vi "Eurotherm set.vi"(8 "error in":errorcluster, 10 "SP&CRC":u8[](array[numeric])=[65, 32, 0, 0, 133, 120], 11 "Addressing":u8[](array[numeric])=[1, 16, 128, 52, 0, 2, 4]) -> (0 "error out":errorcluster)   [LabVIEW 2011]
uses:
  <vilib>/rvi/eio/common/nirviEmuTemplateMethod_errors.vi
  <vilib>/eio/EIOMethodNode/EIOMethodNode.xnode
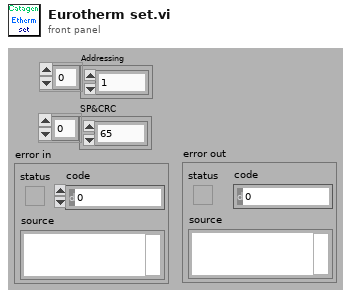
[diagram p1: front panel]
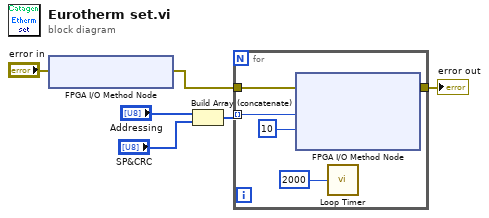
[diagram p0: block diagram]
diagram:
  n1 = xnode "FPGA I/O Method Node"("error in"="error in") -> ("error out"=w3:errorcluster)  [unwired: 1 in, 1 out]
  n2 = Build Array (concatenate)("Addressing", "SP&CRC") -> (w5:u8[])
  n3 = for {
    tunnel: w5 -> [w10] mode=indexing
    tunnel: w3 -> [w8]
    tunnel: [w7] -> w1
    n4 = xnode "FPGA I/O Method Node"("error in"=w8, "Data"=w10, "Timeout (ms)"=10) -> ("error out"=w7:errorcluster)  [unwired: 1 in, 2 out]
    n5 = call "Loop Timer"("Count(uSec)"=u32 2000 ("Count(Ticks)")) -> ()  [unwired: 1 out]
  }
  "error out" <- w1
